vi "Condition Tag Name.vi"(11 "tag in":string) -> (3 "tag out":string)   [LabVIEW 2023, in "uLib.lvlib" / "uData.lvclass"]
doc: "Condition the tag name, to make it case insensitive and handle special use cases such as blank strings."
uses:
  uData.lvclass
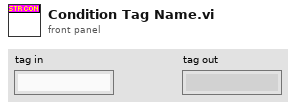
[diagram p1: front panel]
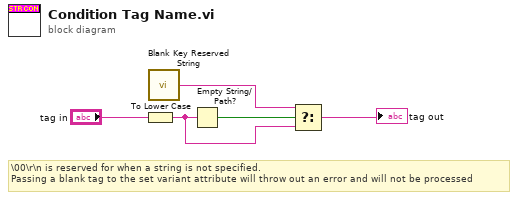
[diagram p0: block diagram]
diagram:
  # "\\00\\r\\n is reserved for when a string is not specified.\nPassing a blank tag to the set variant attribute will throw out an error and will not be processed"
  n1 = To Lower Case(string="tag in") -> (all lower case string=w2:string)
  n2 = call "Blank Key Reserved String.vi"() -> ("Reserved characters"=w1:string)
  n3 = Empty String/Path?(string/path=w2) -> (empty?=w3:bool)
  n4 = Select(t=w1, s=w3, f=w2) -> (s? t:f=→"tag out":string)
